vi "Text Source.vi"(8 "Error In":errorcluster) -> (0 "Error Out":errorcluster)   [LabVIEW 2018, in "Tests.lvlib" / "Nodes.lvlib"]
uses:
  Nodes.lvlib
  src/Toolkit/Low-Level/Nodes/Text/Text.lvclass
  <vilib>/addons/_JKI Toolkits/Caraya/classes/Test/Test.lvclass
  <vilib>/addons/_JKI Toolkits/Caraya/classes/Assert/Assert.lvclass
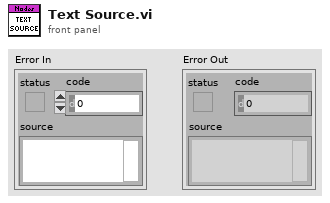
[diagram p1: front panel]
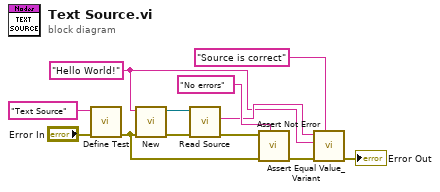
[diagram p0: block diagram]
diagram:
  w1 = "Hello World!" ("Key")
  n1 = call <vilib>:"Define Test.vi"("error in (no error)"="Error In", "Label (VI Title)"="Text Source") -> ("error out"=w4:errorcluster)  [unwired: 9 in]
  n2 = call "New.vi"("Error In"=w4, "Content"=w1) -> ("Error Out"=w3:errorcluster, "Text"=w2:refnum<class "Text.lvclass">)  [unwired: 8 in]
  n3 = call-dynamic "Read Source.vi"("Error In"=w3, "Node In"=w2) -> ("Error Out"=w8:errorcluster, "Source"=w7:string)  [unwired: 7 in, 1 out]
  n4 = call <vilib>:"Assert Not Error.vi"("Label"="No errors", "error in (no error)"=w4, "Not Error?"=w8) -> ("error out"=w10:errorcluster)  [unwired: 8 in]
  n5 = call <vilib>:"Assert Equal Value_Variant.vi"("Label"="Source is correct", "error in (no error)"=w10, "Y"=w1, "X"=w7) -> ("error out"=→"Error Out":errorcluster)  [unwired: 7 in]
